vi "Intro_EV3.vi"   [LabVIEW 2012]
uses:
  SubVIs/LVPresent_Globals.vi
  <vilib>/zip/NI_Unzip.lvlib
panel:
  # "LEGO Mindstorms EV3: Getting Started\n\nThe goal of this book is to get you started in LabVIEW with the EV3 - you will need 1 EV3 kit - please build a  car (directions in the LEGO MINDSTORMS EV3 Manual, or you can just build your own), making sure to connect the motors to ports A and D, or B and C."
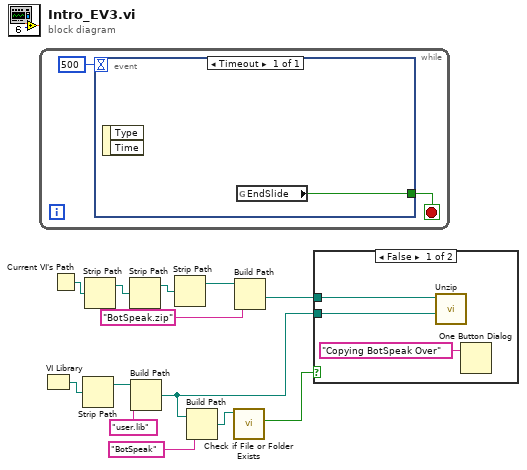
[diagram p0: block diagram]
diagram:
  n1 = while {
    stop <- w15 stop-if-true
    n2 = event shown="[0] Timeout" {
      selector: _ -> [_]
      dyn-events: _ -> [_]
      timeout: 500 -> [_]
      tunnel: [w16] -> w15
      event Timeout {
        n3 = event-data() -> ()  [unwired: 1 in, 2 out]
        n4 = global read "LVPresent_Globals.vi" "EndSlide"() -> (w16:bool)
      }
    }
  }
  n5 = VI Library() -> (path=w9:path)
  n6 = Current VI's Path() -> (path=w13:path)
  n7 = Strip Path(path=w9) -> (stripped path=w7:path)  [unwired: 1 out]
  n8 = Strip Path(path=w13) -> (stripped path=w12:path)  [unwired: 1 out]
  n9 = Strip Path(path=w12) -> (stripped path=w2:path)  [unwired: 1 out]
  n10 = Build Path(base path=w7, name or relative path="user.lib") -> (appended path=w6:path)
  n11 = Strip Path(path=w2) -> (stripped path=w1:path)  [unwired: 1 out]
  n12 = Build Path(base path=w6, name or relative path="BotSpeak") -> (appended path=w4:path)
  n13 = call <vilib>:"Check if File or Folder Exists.vi"("path"=w4) -> ("file or folder exists?"=w3:bool)  [unwired: 8 in, 2 out]
  n14 = Build Path(base path=w1, name or relative path="BotSpeak.zip") -> (appended path=w10:path)
  n15 = case shown="False" w3 {
    tunnel: w10 -> [w19 _]
    tunnel: w6 -> [w18 _]
    frame False {
      n16 = call <vilib>:"Unzip.vi"("Target directory (same as Zip file if empty)"=w18, "Zip file"=w19) -> ()  [unwired: 7 in, 3 out]
      n17 = One Button Dialog(message="Copying BotSpeak Over") -> ()  [unwired: 1 in, 1 out]
    }
    frame True {
    }
  }
